vi "密码.vi"(4 "字符串 2":string="niubi", 5 "密码":string, 6 "用户名":string, 7 "字符串":string="cuger") -> (3 "x与y？":bool)   [LabVIEW 2018]
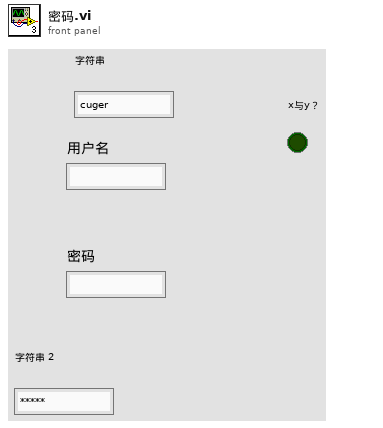
[diagram p1: front panel]
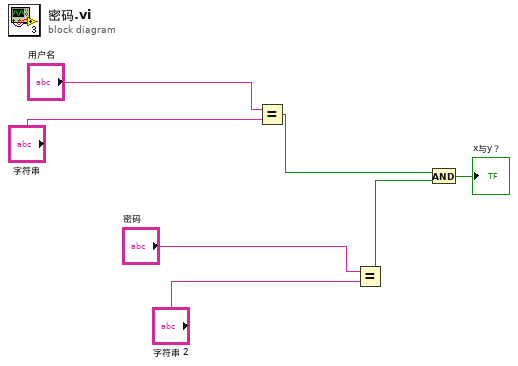
[diagram p0: block diagram]
diagram:
  n1 = Equal?(x="用户名", y="字符串") -> (x = y?=w5:bool)
  n2 = Equal?(x="密码", y="字符串 2") -> (x = y?=w4:bool)
  n3 = And(x=w5, y=w4) -> (x .and. y?=→"x与y？":bool)
